vi "n x n Smoothen Array (SGL) v3.vi"(4 "Average":bool caption="Average (F)", 6 "Threshold Low":sgl=-inf, 7 "Threshold High":sgl=inf, 8 "Error In":errorcluster, 9 "Kernel Size":i32=1, 10 "Kernel Type":T1, 11 "Array in":sgl[][](array[numeric])) -> (0 "Error Out":errorcluster, 1 "Valid?":bool[][](array[boolean]), 3 "Array out":sgl[][](array[numeric]))   [LabVIEW 2021, in "Arrays.lvlib"]
uses:
  Arrays.lvlib
  Kernel Type.ctl
  d0ebc029-cbaa-4c82-a58c-923c59c440da.vi
  b80d5e79-a0c8-46e2-aba9-3d60e0093a16.vi
  Replace NaN by 0 (2D SGL).vi/df975b44-f6c5-4554-af30-980613d33749.vi
  Time/Time.lvlib
panel:
  out "elapsed (relative) seconds":dbl
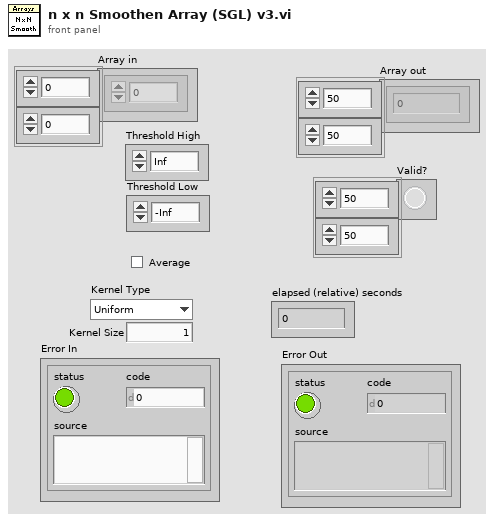
[diagram p1: front panel]
types:
  T1 = typedef "Arrays.lvlib/Kernel Type.ctl" = enum16{"Uniform", "Bilinear", "Gaussian"}
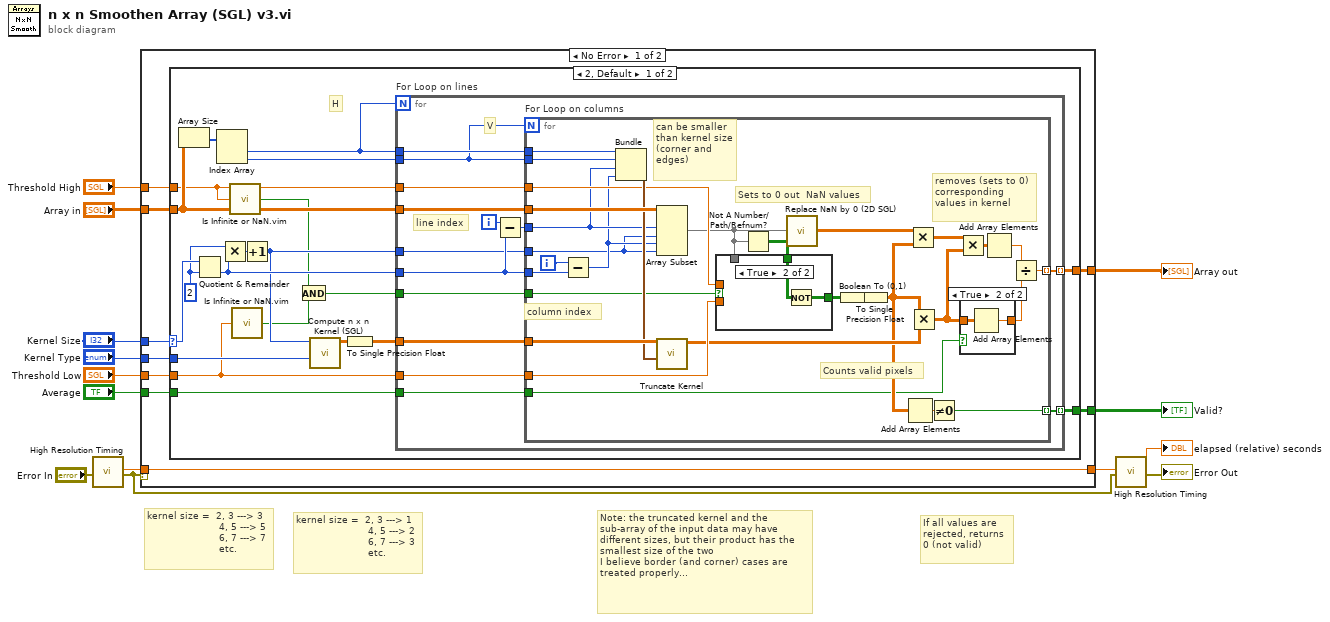
[diagram p0: block diagram]
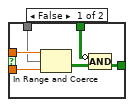
[diagram p2: hidden frame]
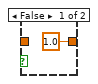
[diagram p3: hidden frame]
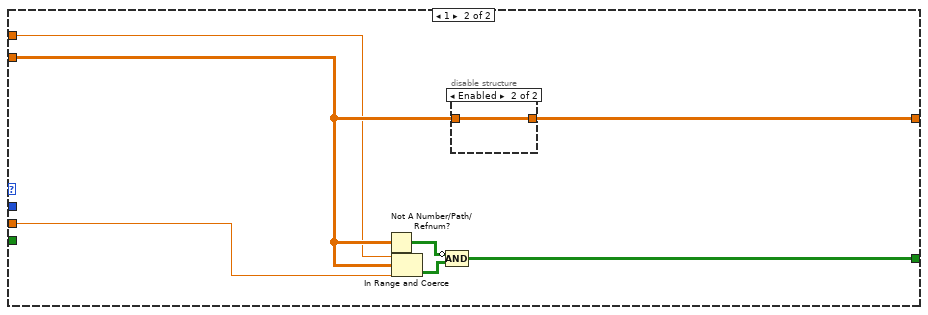
[diagram p4: hidden frame]
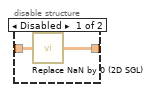
[diagram p5: hidden frame]
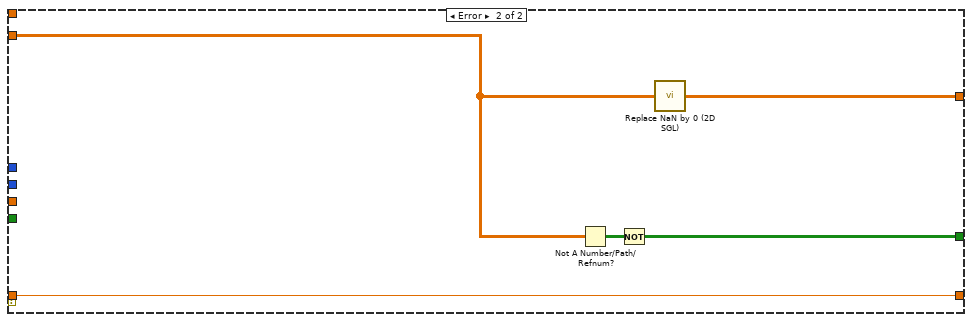
[diagram p6: hidden frame]
diagram:
  # "Note: the truncated kernel and the sub-array of the input data may have different sizes, but their product has the smallest size of the two\nI believe border (and corner) cases are treated properly..."
  # "kernel size =  2, 3 ---> 3\n                        4, 5 ---> 5\n                        6, 7 ---> 7\n                        etc."
  # "kernel size =  2, 3 ---> 1\n                        4, 5 ---> 2\n                        6, 7 ---> 3\n                        etc."
  # "If all values are rejected, returns 0 (not valid)"
  n1 = call "High Resolution Timing.vi"("Error In"="Error In") -> ("elapsed (relative) seconds"=w3:dbl, "Error Out"=w4:errorcluster)  [unwired: 16 in, 1 out]
  n2 = case shown="No Error" w4 {
    tunnel: "Array in" -> [w23 w110]
    tunnel: "Kernel Size" -> [w22 _]
    tunnel: [w21 w111] -> w13
    tunnel: "Threshold Low" -> [w20 _]
    tunnel: "Threshold High" -> [w19 _]
    tunnel: [w18 w109] -> w12
    tunnel: [w15 w108] -> w1
    tunnel: "Kernel Type" -> [w17 _]
    tunnel: "Average" -> [w16 _]
    tunnel: w3 -> [w15 w108]
    frame No Error {
      n3 = case shown="2, Default" w22 {
        selector: w22 -> [w41 _]
        tunnel: w23 -> [w30 w101]
        tunnel: [w37 w104] -> w21
        tunnel: w20 -> [w28 w99]
        tunnel: w19 -> [w27 w100]
        tunnel: [w33 w102] -> w18
        tunnel: w17 -> [w32 _]
        tunnel: w16 -> [w29 _]
        frame 2, Default {
          w35 = 2 ("y")
          # "H"
          n4 = Array Size(array=w30) -> (size(s)=w43:i32[])
          n5 = Quotient & Remainder(x=w41, y=w35) -> (floor(x/y)=w36:i32)  [unwired: 1 out]
          n6 = Index Array(array=w43) -> (element #1=w39:i32, element #2=w42:i32)  [unwired: 2 in]
          n7 = Multiply(x=w35, y=w36) -> (x*y=w34:i32)
          n8 = call "Is Infinite or NaN.vim"("Number"=w27) -> ("Is NaN or Inf?"=w25:bool)  [unwired: 8 in]
          n9 = call "Is Infinite or NaN.vim"("Number"=w28) -> ("Is NaN or Inf?"=w26:bool)  [unwired: 8 in]
          n10 = Increment(x=w34) -> (x+1=w31:i32)
          n11 = And(x=w25, y=w26) -> (x .and. y?=w24:bool)
          n12 = call "Compute n x n Kernel (SGL).vi"("Kernel Type"=w32, "Kernel Size"=w31) -> ("Kernel"=w40:sgl[][])  [unwired: 9 in]
          n13 = To Single Precision Float(number=w40) -> (single precision float=w38:sgl[][])
          n14 = for "For Loop on lines" {
            N: w39 -> [_]
            tunnel: w30 -> [w57]
            tunnel: w42 -> [w50]
            tunnel: w36 -> [w54]
            tunnel: w31 -> [w53]
            tunnel: w38 -> [w52]
            tunnel: w39 -> [w51]
            tunnel: [w49] -> w37 mode=indexing
            tunnel: w28 -> [w48]
            tunnel: w27 -> [w47]
            tunnel: [w46] -> w33 mode=indexing
            tunnel: w29 -> [w45]
            tunnel: w24 -> [w44]
            i -> [w56]
            # "line index"
            # "V"
            n15 = Subtract(x=w56, y=w54) -> (x-y=w55:i32)
            n16 = for "For Loop on columns" {
              N: w50 -> [_]
              tunnel: w57 -> [w86]
              tunnel: w55 -> [w65]
              tunnel: w54 -> [w84]
              tunnel: w53 -> [w63]
              tunnel: w52 -> [w78]
              tunnel: w51 -> [w83]
              tunnel: w50 -> [w82]
              tunnel: [w79] -> w49 mode=indexing
              tunnel: w48 -> [w74]
              tunnel: w47 -> [w75]
              tunnel: [w69] -> w46 mode=indexing
              tunnel: w45 -> [w62]
              tunnel: w44 -> [w58]
              i -> [w85]
              # "Counts valid pixels"
              # "column index"
              # "can be smaller than kernel size (corner and edges)"
              # "removes (sets to 0) corresponding values in kernel"
              # "Sets to 0 out  NaN values"
              n17 = Subtract(x=w85, y=w84) -> (x-y=w64:i32)
              n18 = Bundle(w83, w82, w65, w64) -> (w77:cluster{i32, i32, i32, i32})  [unwired: 1 in]
              n19 = Array Subset(array=w86, index (row)=w65, length (row)=w63, index (col)=w64, length (col)=w63) -> (w68:sgl[][])
              n20 = call "Truncate Kernel.vi"("Array Element Parameters"=w77, "Kernel in"=w78) -> ("Kernel out"=w71:sgl[][])  [unwired: 9 in]
              n21 = Not A Number/Path/Refnum?(number/path/refnum=w68) -> (NaN/Path/Refnum?=w59:bool[][])
              n22 = case shown="True" w58 {
                tunnel: w75 -> [w92 _]
                tunnel: w74 -> [w91 _]
                tunnel: w68 -> [w90 _]
                tunnel: [w88 w93] -> w60
                tunnel: w59 -> [w87 w94]
                frame False {
                  n23 = In Range and Coerce(upper limit=w92, x=w90, lower limit=w91) -> (In Range?=w89:bool[][])  [unwired: 1 out]
                  n24 = Compound Arithmetic op=AND(invert w87, w89) -> (w88:bool[][])
                }
                frame True {
                  n25 = Not(x=w94) -> (.not. x?=w93:bool[][])
                }
              }
              n26 = call "Replace NaN by 0 (2D SGL).vi"("Array in"=w68) -> ("Array out"=w66:sgl[][])  [unwired: 8 in]
              n27 = Boolean To (0,1)(Boolean=w60) -> (0, 1=w61:i16[][])
              n28 = To Single Precision Float(number=w61) -> (single precision float=w67:sgl[][])
              n29 = Add Array Elements(numeric array=w67) -> (sum=w72:sgl)
              n30 = Multiply(x=w66, y=w67) -> (x*y=w73:sgl[][])
              n31 = Multiply(x=w67, y=w71) -> (x*y=w70:sgl[][])
              n32 = Not Equal To 0?(x=w72) -> (x != 0?=w69:bool)
              n33 = Multiply(x=w73, y=w70) -> (x*y=w76:sgl[][])
              n34 = case shown="True" w62 {
                tunnel: [sgl 1.0 w97] -> w80
                tunnel: w70 -> [_ w96]
                frame False {
                }
                frame True {
                  n35 = Add Array Elements(numeric array=w96) -> (sum=w97:sgl)
                }
              }
              n36 = Add Array Elements(numeric array=w76) -> (sum=w81:sgl)
              n37 = Divide(x=w81, y=w80) -> (x/y=w79:sgl)
            }
          }
        }
        frame 1 {
          n38 = Not A Number/Path/Refnum?(number/path/refnum=w101) -> (NaN/Path/Refnum?=w103:bool[][])
          n39 = In Range and Coerce(upper limit=w100, x=w101, lower limit=w99) -> (In Range?=w98:bool[][])  [unwired: 1 out]
          n40 = Compound Arithmetic op=AND(invert w103, w98) -> (w102:bool[][])
          n41 = disable-structure shown="Enabled" {
            disable-tunnel: [w106 w107] -> w104
            disable-tunnel: w101 -> [w105 w107]
            frame Disabled {
              n42 = call "Replace NaN by 0 (2D SGL).vi"("Array in"=w105) -> ("Array out"=w106:sgl[][])  [unwired: 8 in]
            }
            frame Enabled {
            }
          }
        }
      }
    }
    frame Error {
      n43 = Not A Number/Path/Refnum?(number/path/refnum=w110) -> (NaN/Path/Refnum?=w112:bool[][])
      n44 = Not(x=w112) -> (.not. x?=w109:bool[][])
      n45 = call "Replace NaN by 0 (2D SGL).vi"("Array in"=w110) -> ("Array out"=w111:sgl[][])  [unwired: 8 in]
    }
  }
  "Array out" <- w13
  "Valid?" <- w12
  n46 = call "High Resolution Timing.vi"("relative seconds (NaN)"=w1, "Error In"=w4) -> ("elapsed (relative) seconds"=→"elapsed (relative) seconds":dbl, "Error Out"=→"Error Out":errorcluster)  [unwired: 15 in, 1 out]
